vi "SDCP FTOR Encode.vi"(3 "error in (no error)":errorcluster, 5 "?":T1) -> (0 "error out":errorcluster, 1 "FTOR2 frame":u8[](array[numeric]), 2 "FTOR1 frame":u8[](array[numeric]))   [LabVIEW 2020]
uses:
  Typedefs/SDCP FTOR params.ctl
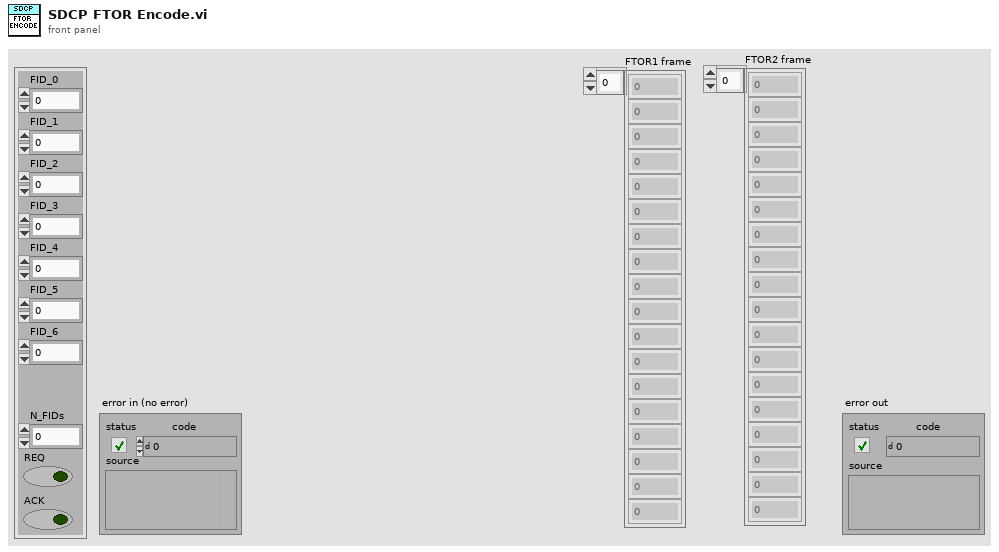
[diagram p1: front panel]
types:
  T1 = typedef "SDCP FTOR params.ctl" = cluster{"FID_0":i32, "FID_1":i32, "FID_2":i32, "FID_3":i32, "FID_4":i32, "FID_5":i32, "FID_6":i32, "N_FIDs":i32, "REQ":bool, "ACK":bool}
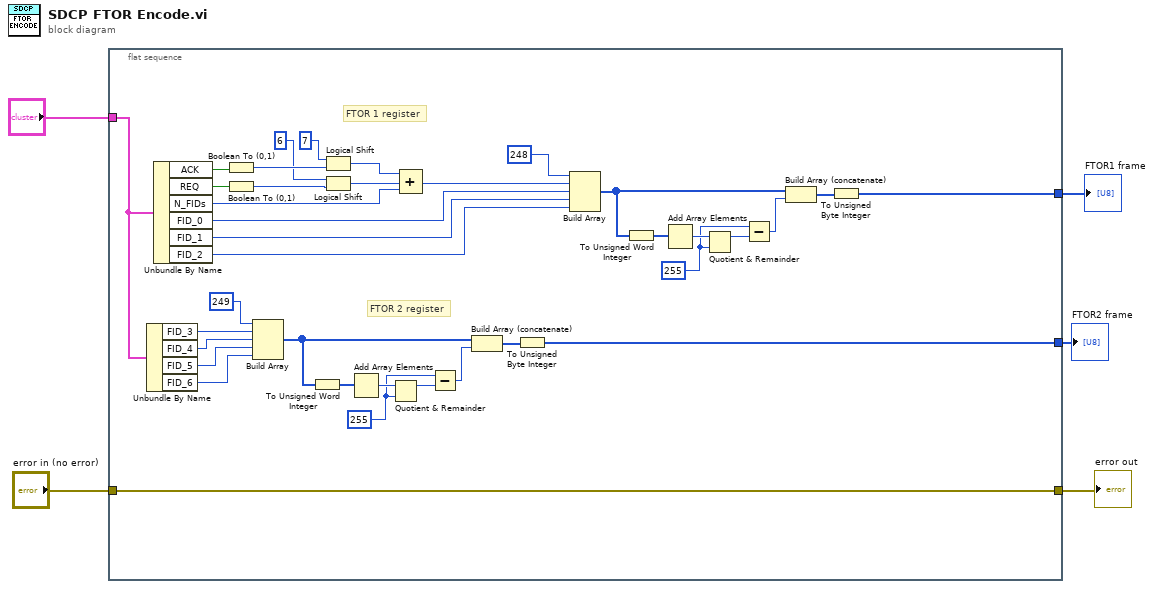
[diagram p0: block diagram]
diagram:
  n1 = flat-sequence {
    tunnel: [w21] -> w5
    tunnel: "?" -> [w20]
    tunnel: [w7] -> w3
    tunnel: "error in (no error)" -> [w6]
    tunnel: [w6] -> w1
    frame #0 {
      w11 = u16 255 ("y")
      w24 = u16 255 ("y")
      # "FTOR 2 register"
      # "FTOR 1 register"
      n2 = Unbundle By Name(w20) -> ("FID_3"=w19:i32, "FID_4"=w18:i32, "FID_5"=w17:i32, "FID_6"=w16:i32)
      n3 = Unbundle By Name(w20) -> ("ACK"=w42:bool, "REQ"=w41:bool, "N_FIDs"=w36:i32, "FID_0"=w32:i32, "FID_1"=w31:i32, "FID_2"=w30:i32)
      n4 = Boolean To (0,1)(Boolean=w42) -> (0, 1=w40:i16)
      n5 = Boolean To (0,1)(Boolean=w41) -> (0, 1=w38:i16)
      n6 = Build Array(249 ("element"), w19, w18, w17, w16) -> (w8:i32[])
      n7 = To Unsigned Word Integer(number=w8) -> (unsigned 16bit integer=w14:u16[])
      n8 = Logical Shift(y=i16 7, x=w40) -> (x << y=w34:i16)
      n9 = Logical Shift(y=i16 6, x=w38) -> (x << y=w35:i16)
      n10 = Add Array Elements(numeric array=w14) -> (sum=w13:u16)
      n11 = Quotient & Remainder(x=w13, y=w11) -> (x-y*floor(x/y)=w12:u16)  [unwired: 1 out]
      n12 = Compound Arithmetic op=ADD(w34, w35, w36) -> (w33:i32)
      n13 = Subtract(x=w11, y=w12) -> (x-y=w10:u16)
      n14 = Build Array (concatenate)(w8, w10) -> (w9:i32[])
      n15 = To Unsigned Byte Integer(number=w9) -> (unsigned 8bit integer=w7:u8[])
      n16 = Build Array(248 ("element"), w33, w32, w31, w30) -> (w26:i32[])
      n17 = To Unsigned Word Integer(number=w26) -> (unsigned 16bit integer=w28:u16[])
      n18 = Add Array Elements(numeric array=w28) -> (sum=w27:u16)
      n19 = Quotient & Remainder(x=w27, y=w24) -> (x-y*floor(x/y)=w25:u16)  [unwired: 1 out]
      n20 = Subtract(x=w24, y=w25) -> (x-y=w23:u16)
      n21 = Build Array (concatenate)(w26, w23) -> (w22:i32[])
      n22 = To Unsigned Byte Integer(number=w22) -> (unsigned 8bit integer=w21:u8[])
    }
  }
  "error out" <- w1
  "FTOR1 frame" <- w5
  "FTOR2 frame" <- w3
